vi "Read Command.vi"(11 "Generator Data in":T1) -> (3 "Generator Data out":T1)   [LabVIEW 2016]
uses:
  Typedefs/Generator Data Cluster.ctl
  <vilib>/rvi/interface/RandomDataEmulation/niFpgaRandomDataHandleErrors.vi
  <vilib>/rvi/Emulation/niFpgaEmulationIsFPGAContextNoSignature.vi
  <vilib>/rvi/DataTransferAndStorage/Container/Common/niFpgaContainerGetUniqueNameForEmu.vi
  <vilib>/rvi/Memory/Memory_Emulation/niFpgaMemoryEmulationCacheClearOnFirstRun.vi
  <vilib>/rvi/Memory/Memory_Emulation/nirvimemoryEmulationManagerCache_MakeExclusive.vi
  <vilib>/rvi/Memory/Memory_Emulation/niFpgaMemoryEmulationValidateCache.vi
  <vilib>/rvi/Memory/Memory_Emulation/nirvimemoryEmulationManagerCache_InsertValue.vi
  <vilib>/Utility/error.llb/Clear Errors.vi
  <vilib>/rvi/Memory/Memory_Emulation/nirvimemoryEmulationManagerCache_ReleaseExclusive.vi
  <vilib>/rvi/Memory/Memory_Emulation/nirvimemoryEmulationManagerCache_GetValue.vi
  <vilib>/rvi/Memory/Memory_Emulation/nirvimemoryEmulationManagerCache_SetValue.vi
  <vilib>/rvi/Emulation/niFpgaProcessEmulError.vi
  <vilib>/rvi/Emulation/niFpgaSctlEmulationGetInTimedLoop.vi
  <vilib>/rvi/DataTransferAndStorage/Container/XNode/niFpgaContainer.xnode
  <vilib>/rvi/interface/RandomDataEmulation/nirviRandomDataFpgaReadWriteTemplate.vi
  <vilib>/rvi/DataTransferAndStorage/Register/Emulation/niFpgaRegisterEmulation.vi
  Host/Typedefs/IO Buffer Operation.ctl
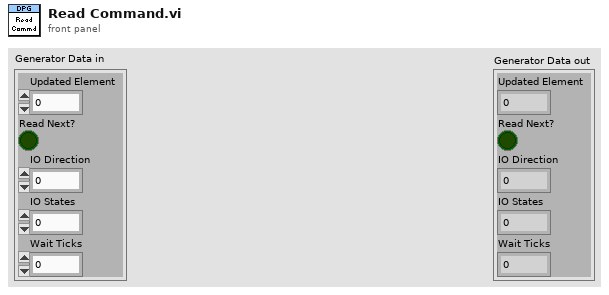
[diagram p1: front panel]
types:
  T1 = typedef "Generator Data Cluster.ctl" = cluster{"Updated Element":u64, "Read Next?":bool, "IO Direction":u32, "IO States":u32, "Wait Ticks":u32}
  T2 = typedef "IO Buffer Operation.ctl" = enum16{"Initialize", "Write IO Data_Rd", "Read IO Data_Rd", "Write IO Data_Wr", "Read IO Data_Wr", "Write  IO Data_Dir", "Read  IO Data_Dir", "Write Host to Target FIFO", "Read Host to Target FIFO", "Write Target to Host FIFO", "Read Target to Host FIFO", "Write Monitor Enable?", "Read Monitor Enable?", "Close"}
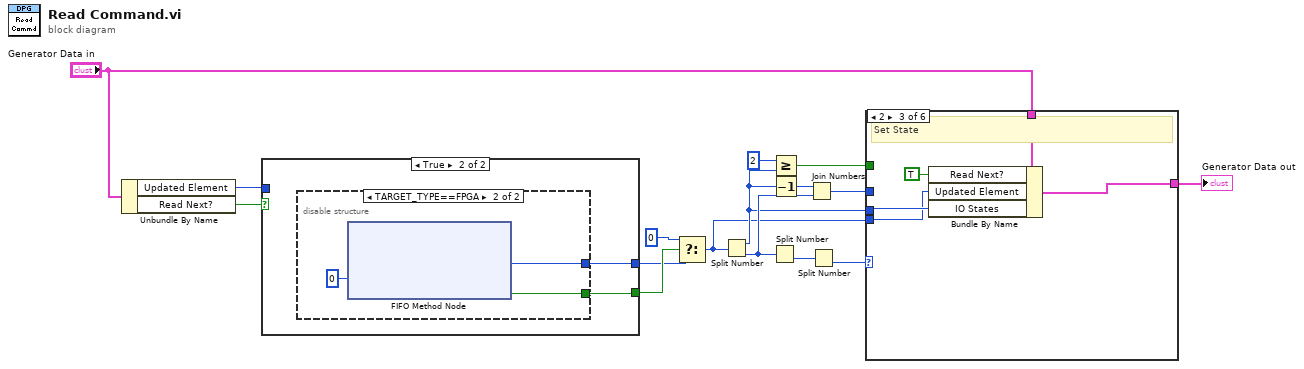
[diagram p0: block diagram]
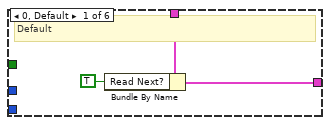
[diagram p2: hidden frame]
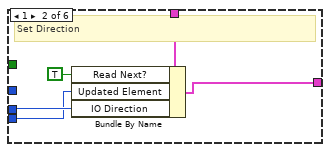
[diagram p3: hidden frame]
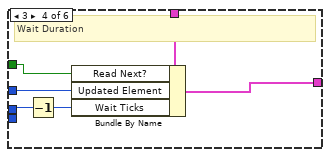
[diagram p4: hidden frame]
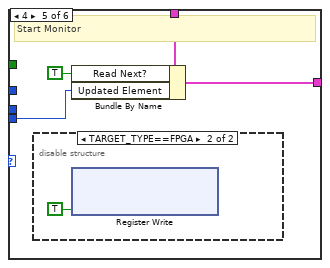
[diagram p5: hidden frame]
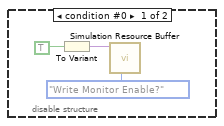
[diagram p6: hidden frame]
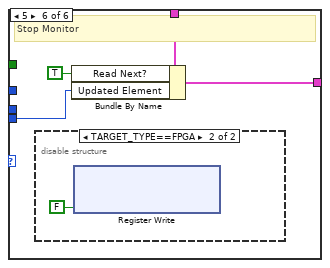
[diagram p7: hidden frame]
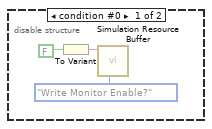
[diagram p8: hidden frame]
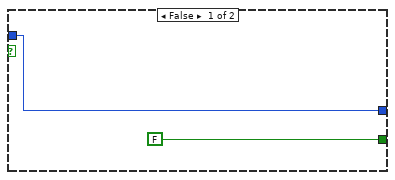
[diagram p9: hidden frame]
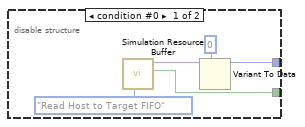
[diagram p10: hidden frame]
diagram:
  n1 = Unbundle By Name("Generator Data in") -> ("Updated Element"=w10:u64, "Read Next?"=w9:bool)
  n2 = case shown="True" w9 {
    tunnel: [w18 w20] -> w14
    tunnel: w10 -> [w18 _]
    tunnel: [FALSE ("Timed Out?") w19] -> w15
    frame False {
    }
    frame True {
      n3 = disable-structure shown="TARGET_TYPE==FPGA" {
        disable-tunnel: [w21 w27] -> w20
        disable-tunnel: [w24 w26] -> w19
        frame condition #0 {
          n4 = call "Simulation Resource Buffer.vi"("IO Buffer Operation"=IO_Buffer_Operation."Read Host to Target FIFO") -> ("Timed Out?"=w24:bool, "Data out"=w23:variant)  [unwired: 8 in, 1 out]
          n5 = Variant To Data(type=u64 0 ("Element"), Variant=w23) -> (data=w21:u64)  [unwired: 1 in, 1 out]
        }
        frame condition #1 (active) {
          n6 = xnode ("FIFO Method Node")("Timeout"=0) -> ("Element"=w27:u64, "Timed Out?"=w26:bool)  [unwired: 1 in, 1 out]
        }
      }
    }
  }
  n7 = Select(t=u64 0, s=w15, f=w14) -> (s? t:f=w1:u64)
  n8 = Split Number(x=w1) -> (hi(x)=w2:u32, lo(x)=w11:u32)
  n9 = Split Number(x=w11) -> (lo(x)=w16:u16)  [unwired: 1 out]
  n10 = Greater Or Equal?(x=u32 2, y=w2) -> (x >= y?=w3:bool)
  n11 = Decrement(x=w2) -> (x-1=w12:u32)
  n12 = Join Numbers(hi=w12, lo=w11) -> ((hi.lo)=w6:u64)
  n13 = Split Number(x=w16) -> (lo(x)=w8:u8)  [unwired: 1 out]
  n14 = case shown="2" w8 {
    tunnel: w2 -> [_ w34 w39 w45 _ _]
    tunnel: "Generator Data in" -> [w31 w36 w41 w47 w51 w59]
    tunnel: w6 -> [_ _ _ w46 _ _]
    tunnel: [w30 w33 w38 w44 w49 w57] -> w5
    tunnel: w3 -> [_ _ _ w42 _ _]
    tunnel: w1 -> [_ w32 w37 _ w48 w56]
    frame 0, Default {
      # "Default"
      n15 = Bundle By Name(cluster=w31, "Read Next?"=TRUE) -> (w30:T1)
    }
    frame 1 {
      # "Set Direction"
      n16 = Bundle By Name(cluster=w36, "Read Next?"=TRUE, "Updated Element"=w32, "IO Direction"=w34) -> (w33:T1)
    }
    frame 2 {
      # "Set State"
      n17 = Bundle By Name(cluster=w41, "Read Next?"=TRUE, "Updated Element"=w37, "IO States"=w39) -> (w38:T1)
    }
    frame 3 {
      # "Wait Duration"
      n18 = Decrement(x=w45) -> (x-1=w43:u32)
      n19 = Bundle By Name(cluster=w47, "Read Next?"=w42, "Updated Element"=w46, "Wait Ticks"=w43) -> (w44:T1)
    }
    frame 4 {
      # "Start Monitor"
      n20 = disable-structure shown="TARGET_TYPE==FPGA" {
        frame condition #0 {
          n21 = To Variant(anything=TRUE ("Read Next?")) -> (Variant=w52:variant)
          n22 = call "Simulation Resource Buffer.vi"("IO Buffer Operation"=IO_Buffer_Operation."Write Monitor Enable?", "Data in"=w52) -> ()  [unwired: 7 in, 3 out]
        }
        frame condition #1 (active) {
          n23 = xnode ("Register Write")("Data"=TRUE) -> ()  [unwired: 1 in, 1 out]
        }
      }
      n24 = Bundle By Name(cluster=w51, "Read Next?"=TRUE, "Updated Element"=w48) -> (w49:T1)
    }
    frame 5 {
      # "Stop Monitor"
      n25 = disable-structure shown="TARGET_TYPE==FPGA" {
        frame condition #0 {
          n26 = To Variant(anything=FALSE ("Read Next?")) -> (Variant=w60:variant)
          n27 = call "Simulation Resource Buffer.vi"("IO Buffer Operation"=IO_Buffer_Operation."Write Monitor Enable?", "Data in"=w60) -> ()  [unwired: 7 in, 3 out]
        }
        frame condition #1 (active) {
          n28 = xnode ("Register Write")("Data"=FALSE) -> ()  [unwired: 1 in, 1 out]
        }
      }
      n29 = Bundle By Name(cluster=w59, "Read Next?"=TRUE, "Updated Element"=w56) -> (w57:T1)
    }
  }
  "Generator Data out" <- w5
